vi "Pcre2SubstringFromSubjectByOffsets (s).vi"(9 "OffsetPastMatch":i32, 10 "MatchOffset":i32, 11 "Subject":string) -> (2 "Substring":string)   [LabVIEW 2021, in "libpcre2-8.lvlib"]
uses:
  libpcre2-8.lvlib
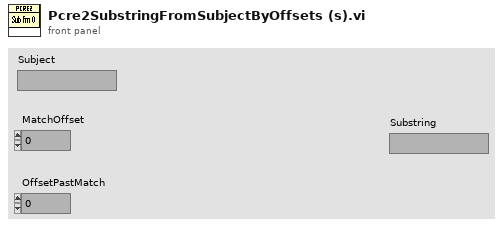
[diagram p1: front panel]
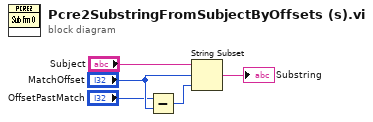
[diagram p0: block diagram]
diagram:
  n1 = Subtract(x="OffsetPastMatch", y="MatchOffset") -> (x-y=w3:i32)
  n2 = String Subset(string="Subject", offset (0)="MatchOffset", length (rest)=w3) -> (substring=→"Substring":string)
